vi "DelayDisplay.vi"() -> ()   [LabVIEW 2022 SP3]
uses:
  <vilib>/Utility/file.llb/Write To Spreadsheet File (DBL).vi
panel:
  out "Intensity Graph":dbl[][](graph)
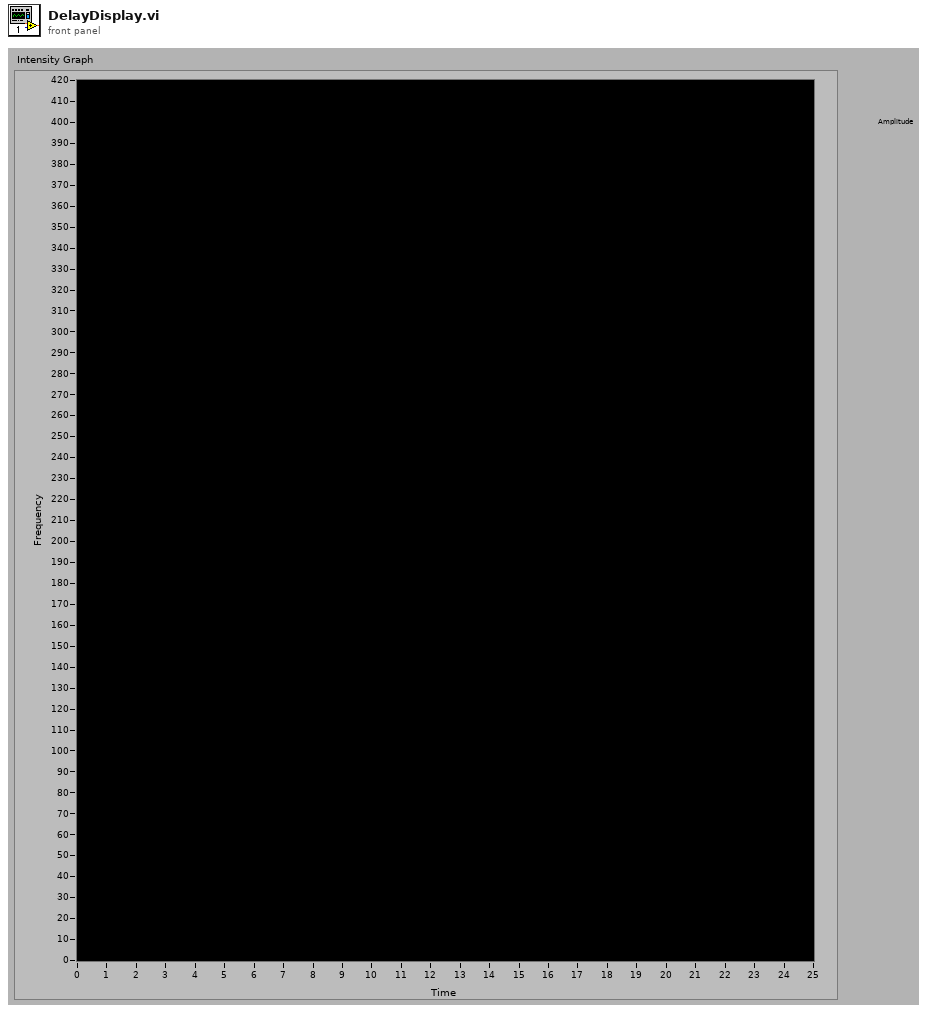
[diagram p1: front panel]
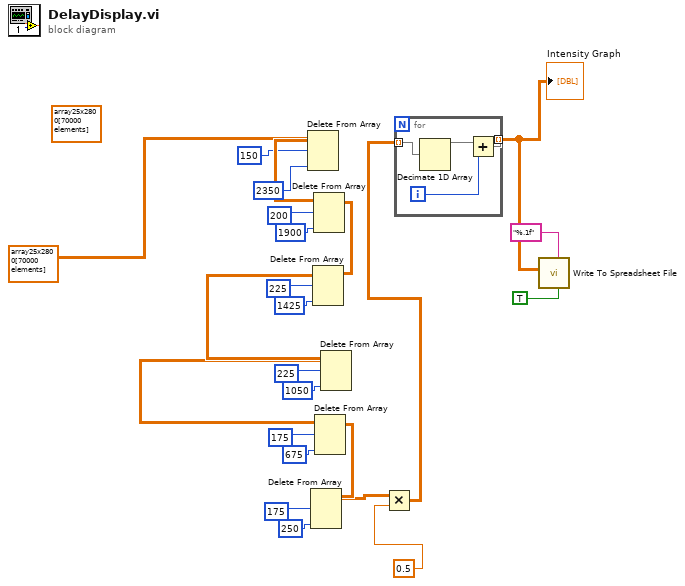
[diagram p0: block diagram]
diagram:
  (unwired) dbl[][] array25x2800[70000 elements] ("Intensity Graph")
  n1 = Delete From Array(array=dbl[][] array25x2800[70000 elements] ("Intensity Graph"), length=150, index (col)=2350 ("index (row)")) -> (array with subset deleted=w23:dbl[][])  [unwired: 1 in, 1 out]
  n2 = Delete From Array(array=w23, length=200, index (col)=1900 ("index (row)")) -> (array with subset deleted=w17:dbl[][])  [unwired: 1 in, 1 out]
  n3 = Delete From Array(array=w17, length=225, index (col)=1425 ("index (row)")) -> (array with subset deleted=w14:dbl[][])  [unwired: 1 in, 1 out]
  n4 = Delete From Array(array=w14, length=225, index (col)=1050 ("index (row)")) -> (array with subset deleted=w9:dbl[][])  [unwired: 1 in, 1 out]
  n5 = Delete From Array(array=w9, length=175, index (col)=675 ("index (row)")) -> (array with subset deleted=w8:dbl[][])  [unwired: 1 in, 1 out]
  n6 = Delete From Array(array=w8, length=175, index (col)=250 ("index (row)")) -> (array with subset deleted=w4:dbl[][])  [unwired: 1 in, 1 out]
  n7 = Multiply(x=w4, y=0.5) -> (x*y=w2:dbl[][])
  n8 = for {
    tunnel: w2 -> [w27] mode=indexing
    tunnel: [w26] -> w3 mode=indexing
    i -> [w28]
    n9 = Decimate 1D Array(w27) -> (w25:dbl[])  [unwired: 3 out]
    n10 = Add(x=w25, y=w28) -> (x+y=w26:dbl[])
  }
  "Intensity Graph" <- w3
  n11 = call-poly <vilib>:"Write To Spreadsheet File.vi"("transpose? (no:F)"=TRUE, "format (%.3f)"="%.1f", "2D data"=w3) -> ()  [unwired: 3 in, 3 out]
